vi "opticPath2freqArray.vi"(1 "b":dbl, 2 "m":dbl, 3 "lamda (nm)":dbl, 4 "camino optico (nm)":dbl[](array[numeric])) -> (0 "freq":dbl[](array[numeric]))   [LabVIEW 2010]
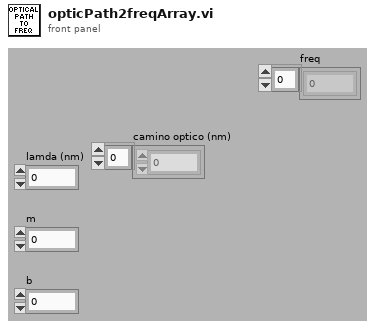
[diagram p1: front panel]
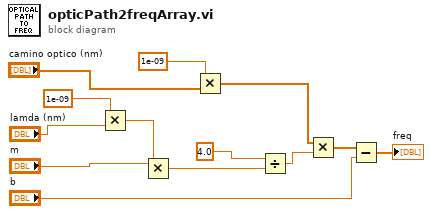
[diagram p0: block diagram]
diagram:
  n1 = Multiply(x=1e-09, y="lamda (nm)") -> (x*y=w6:dbl)
  n2 = Multiply(x="m", y=w6) -> (x*y=w12:dbl)
  n3 = Multiply(x=1e-09, y="camino optico (nm)") -> (x*y=w3:dbl[])
  n4 = Divide(x=4.0, y=w12) -> (x/y=w8:dbl)
  n5 = Multiply(x=w3, y=w8) -> (x*y=w9:dbl[])
  n6 = Subtract(x=w9, y="b") -> (x-y=→"freq":dbl[])
